vi "dvp Vi Get Color Solution Sel Descr.vi"(7 "pbNeedStop":bool, 9 "puCount":u32, 10 "puDefault":u32, 11 "handle":u32) -> (1 "puCount out":u32, 2 "puDefault out":u32, 3 "function return":u32(ring), 5 "pbNeedStop out":bool)   [LabVIEW 2018, in "LabViewDVPCamera.lvlib"]
doc: "LabviewDvp2Api dvpStatus dvpViGetColorSolutionSelDescr(\n dvpHandle handle, \n dvpUint32 *puDefault,\n dvpUint32 *puCount,\n bool *pbNeedStop);"
uses:
  LabViewDVPCamera.lvlib
  LabViewDVPCamera/LabViewDVPCamera.dll
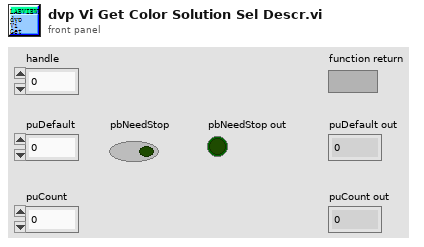
[diagram p1: front panel]
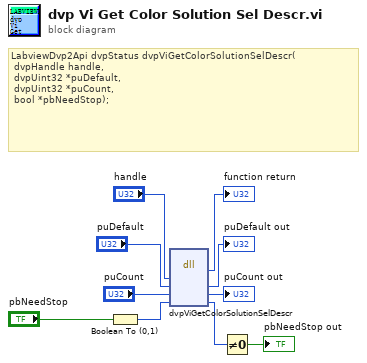
[diagram p0: block diagram]
diagram:
  # "LabviewDvp2Api dvpStatus dvpViGetColorSolutionSelDescr(\n\tdvpHandle handle,   \n\tdvpUint32 *puDefault,\n\tdvpUint32 *puCount,\n\tbool *pbNeedStop);"
  n1 = Boolean To (0,1)(Boolean="pbNeedStop") -> (0, 1=w3:i16)
  n2 = dll-call lib="C:/Program Files (x86)/DVP2 Labview cn 64/Sample/LabViewDVPCamera/LabViewDVPCamera.*" fn="dvpViGetColorSolutionSelDescr"("handle"="handle", "puDefault"="puDefault", "puCount"="puCount", "pbNeedStop"=w3) -> (→"function return":u32, "puDefault"=→"puDefault out":u32, "puCount"=→"puCount out":u32, "pbNeedStop"=w1:u8)  [unwired: 4 in, 2 out]
  n3 = Not Equal To 0?(x=w1) -> (x != 0?=→"pbNeedStop out":bool)
